vi "Test Cryogen Levels.vi"(7 "magarray":T1(array[cluster]), 8 "warningcontN":T2, 9 "warningcontHe":T3, 10 "LNlevel":dbl, 11 "LHelevel":dbl) -> (1 "warnN":bool, 2 "warnHe":bool, 3 "warning":T4)   [LabVIEW 2009, in "Magnet.lvclass"]
uses:
  Magnet.lvclass
  Global/Level Meter.vi
panel:
  # "Off"
  # "On"
  # "Greater"
  # "Less"
  # "Off"
  # "On"
  # "Greater"
  # "Less"
  # "Slow"
  # "Fast"
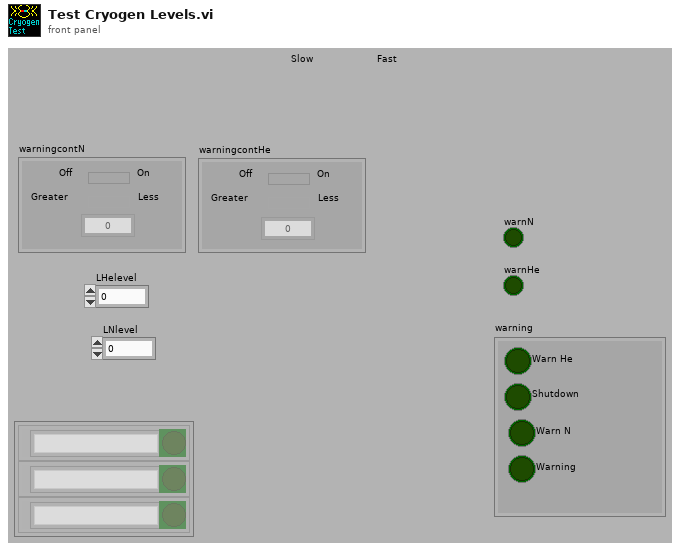
[diagram p1: front panel]
types:
  T1 = cluster{"name":string, "on?":bool, "abbrev":string}[]
  T2 = cluster{"alarmliqN":dbl, "warn?":bool, "lessthan?":bool}
  T3 = cluster{"alarmliqHe":dbl, "warn?":bool, "lessthan?":bool}
  T4 = cluster{"shutdown?":bool, "warnHe":bool, "warnN":bool, "warn":bool}
  T5 = typedef "OxfordAddress.ctl" = cluster{"Com Port":i32, "ISOBUS Address":i32, "GPIB Address":i16, "Communication":enum16{"RS232", "ISOBUS", "GPIB", "Gateway"}}
  T6 = cluster{"Address":T5, "ILM Name":string, "Display Channel":i32[]}
  T7 = typedef "ILMRelayStatus.ctl" = cluster{"Shut down":bool, "Alarm sound":bool, "Alarm state":bool, "Silence prohib":bool, "Relay1 active":bool, "Relay 2 active":bool, "Relay 3 active":bool, "Relay 4 active":bool}
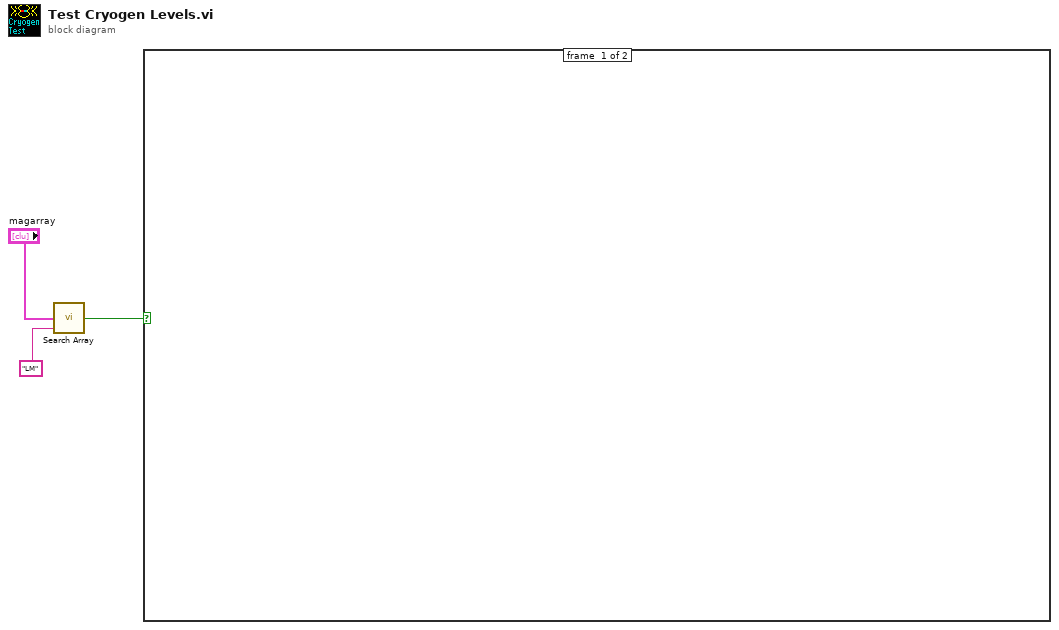
[diagram p0: block diagram]
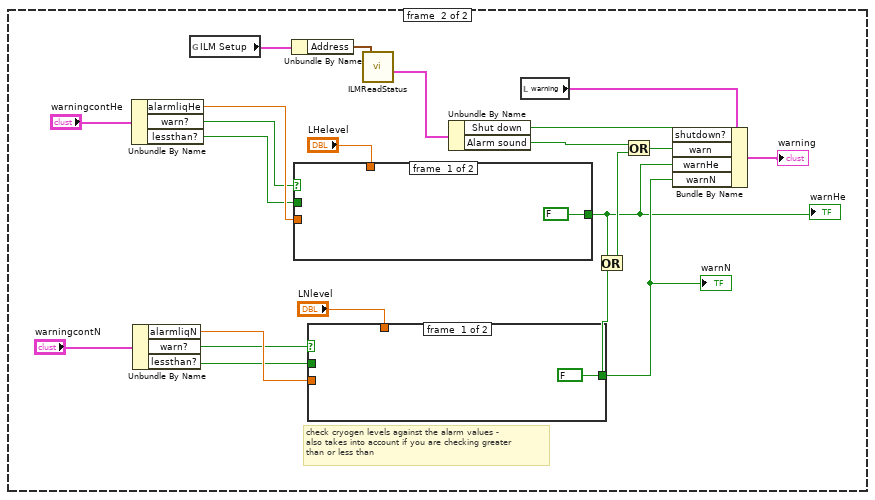
[diagram p2: hidden frame]
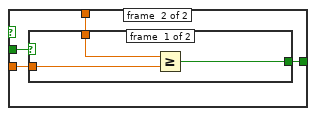
[diagram p3: hidden frame]
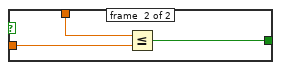
[diagram p4: hidden frame]
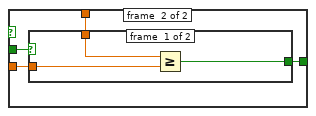
[diagram p5: hidden frame]
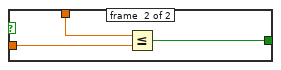
[diagram p6: hidden frame]
diagram:
  n1 = call "Search Array.vi"("abbrev"="LM", "instrarray"="magarray") -> ("on?"=w1:bool)  [unwired: 3 out]
  n2 = case shown="True" w1 {
    frame #0 {
    }
    frame #1 {
      # "check cryogen levels against the alarm values -\nalso takes into account if you are checking greater\nthan or less than"
      n3 = Unbundle By Name("warningcontHe") -> ("alarmliqHe"=w21:dbl, "warn?"=w19:bool, "lessthan?"=w18:bool)
      n4 = Unbundle By Name("warningcontN") -> ("alarmliqN"=w17:dbl, "warn?"=w16:bool, "lessthan?"=w15:bool)
      n5 = global read "Level Meter.vi" "ILM Setup"() -> (w5:T6)
      n6 = Unbundle By Name(w5) -> ("Address"=w4:T5)
      n7 = case shown="True" w19 {
        tunnel: w18 -> [_ w40]
        tunnel: "LHelevel" -> [_ w37]
        tunnel: w21 -> [_ w39]
        tunnel: [FALSE w38] -> w11
        frame #0 {
        }
        frame #1 {
          n8 = case shown="True" w40 {
            tunnel: w39 -> [w42 w45]
            tunnel: [w41 w44] -> w38
            tunnel: w37 -> [w43 w46]
            frame #0 {
              n9 = Greater Or Equal?(x=w43, y=w42) -> (x >= y?=w41:bool)
            }
            frame #1 {
              n10 = Less Or Equal?(x=w46, y=w45) -> (x <= y?=w44:bool)
            }
          }
        }
      }
      "warnHe" <- w11
      n11 = case shown="True" w16 {
        tunnel: w15 -> [_ w29]
        tunnel: "LNlevel" -> [_ w26]
        tunnel: w17 -> [_ w28]
        tunnel: [FALSE w27] -> w14
        frame #0 {
        }
        frame #1 {
          n12 = case shown="True" w29 {
            tunnel: w28 -> [w31 w34]
            tunnel: [w30 w33] -> w27
            tunnel: w26 -> [w32 w35]
            frame #0 {
              n13 = Greater Or Equal?(x=w32, y=w31) -> (x >= y?=w30:bool)
            }
            frame #1 {
              n14 = Less Or Equal?(x=w35, y=w34) -> (x <= y?=w33:bool)
            }
          }
        }
      }
      "warnN" <- w14
      n15 = call "ILMReadStatus.vi"("Instrument address"=w4) -> ("Relay"=w6:T7)  [unwired: 6 out]
      n16 = Unbundle By Name(w6) -> ("Shut down"=w8:bool, "Alarm sound"=w7:bool)
      n17 = local read "warning"() -> (w24:T4)
      n18 = Or(x=w11, y=w14) -> (x .or. y?=w12:bool)
      n19 = Or(x=w7, y=w12) -> (x .or. y?=w13:bool)
      n20 = Bundle By Name(cluster=w24, "shutdown?"=w8, "warn"=w13, "warnHe"=w11, "warnN"=w14) -> (→"warning":T4)
    }
  }
